vi "Relatorio1LabView.vi"() -> ()   [LabVIEW 2019]
uses:
  <vilib>/Instr/_visa.llb/VISA Configure Serial Port (Instr).vi
  <vilib>/express/express analysis/Spectral/Block/exnSpectralBlock spectral measurements RMS poly.vi
  <vilib>/express/express analysis/Spectral/Block/exnSpectralBlock spectral measurements RMS WFM.vi
  <vilib>/express/express analysis/Spectral/XNode/ExpressSpectralMeasurementsBlockNode.xnode
panel:
  out "Análise espectral da onda - FFT (RMS)":cluster{"f0":dbl, "df":dbl, "magnitude":dbl[]}(graph)
  out "Amplitude do sinal (v) x tempo (s):":waveform(dbl)(graph)
  in  "Parar":bool
  out "Número de \nAmostras":u32 caption="Número de Amostras"
  in  "Número de Blocos de Dados":u32=100 min=1 max=50000 step=1
  in  "Frequencia de Amostragem":dbl=75000.0
  in  "VCC":dbl=5.0
  in  "Resolução":i16=8
  in  "COM Port":refnum<visa-resource-name>
  in  "Baudrate":u32=2000000
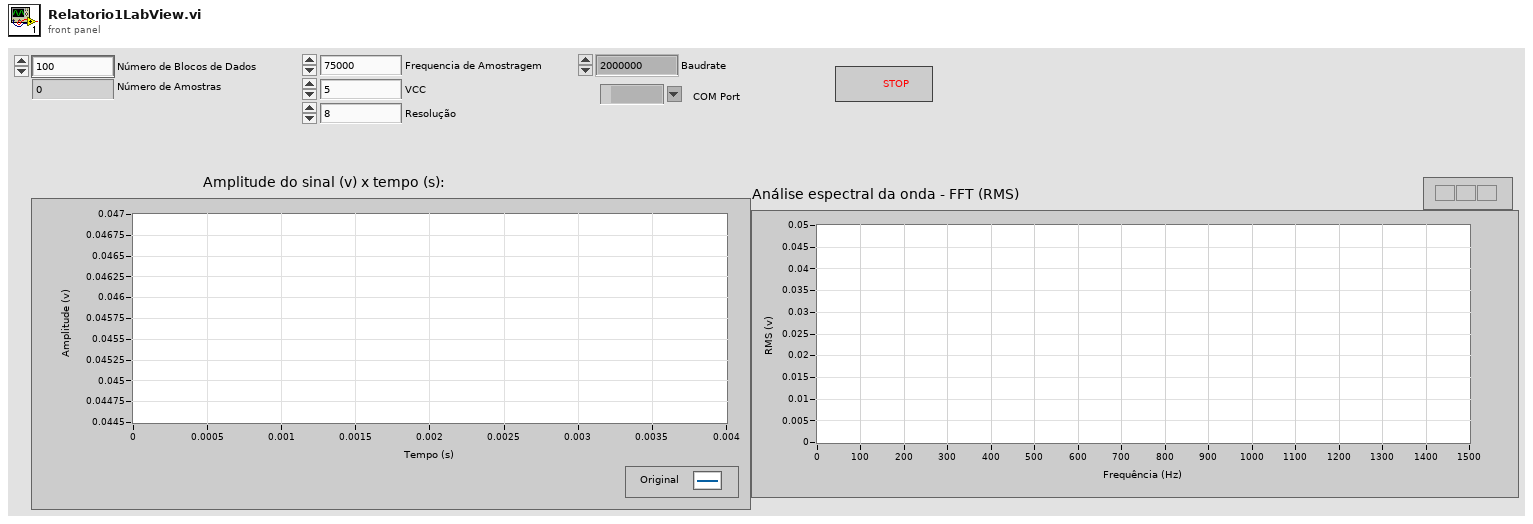
[diagram p1: front panel]
types:
  T1 = cluster{"averaging mode":u16, "weighting mode":u16, "number of averages":u32}
  T2 = cluster{"dB On (F)":bool, "unwrap phase (F)":bool, "convert to degree (F)":bool}
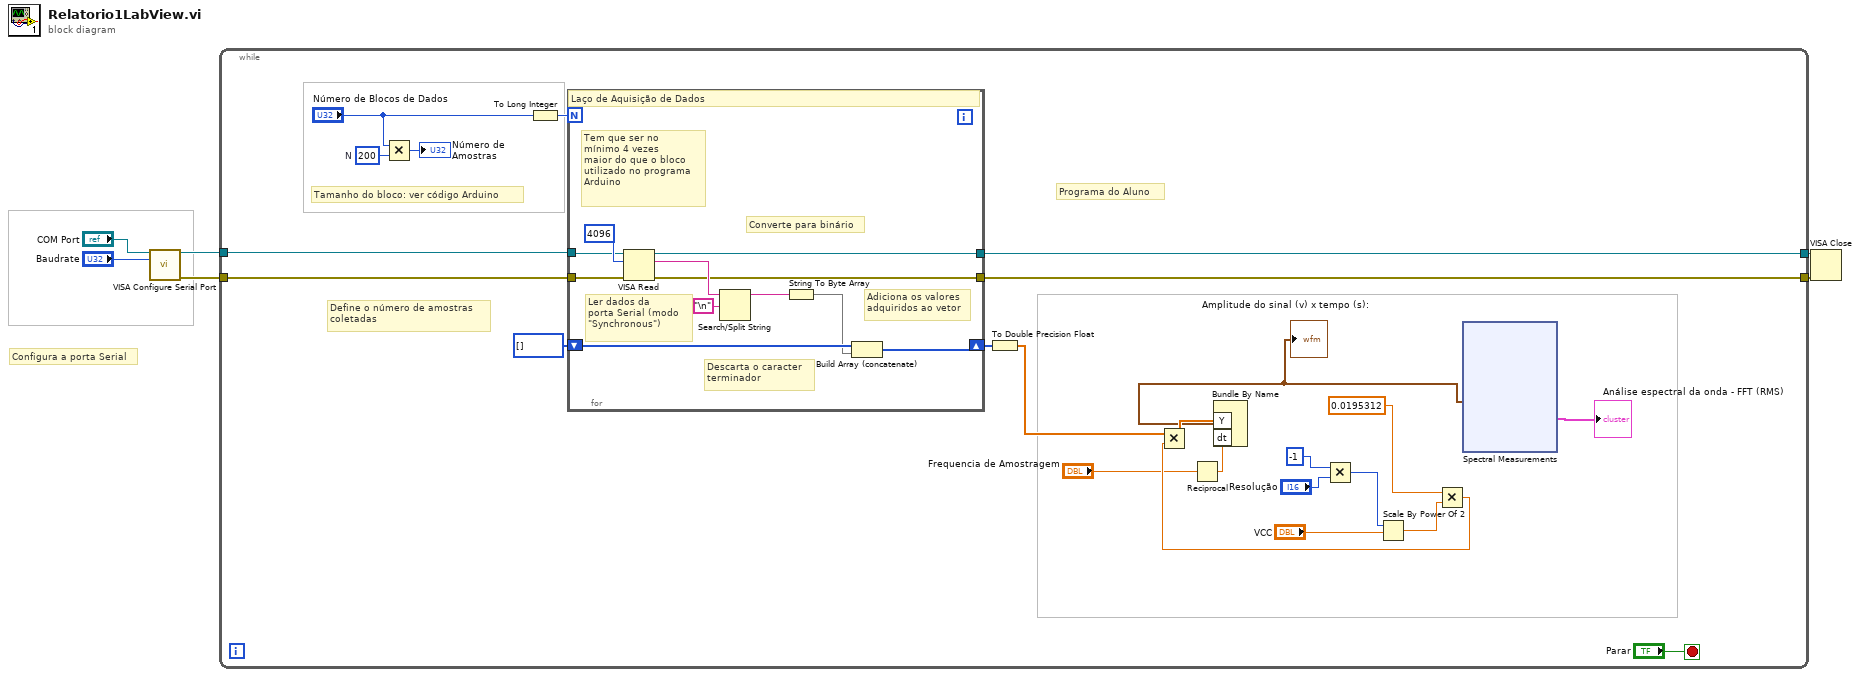
[diagram p0: block diagram]
diagram:
  # "Configura a porta Serial"
  n1 = call-poly "VISA Configure Serial Port"("VISA resource name"="COM Port", "baud rate (9600)"="Baudrate") -> ("VISA resource name out"=w4:refnum<visa-resource-name>, "error out"=w3:errorcluster)  [unwired: 12 in]
  n2 = while {
    tunnel: w4 -> [w30]
    tunnel: w3 -> [w29]
    tunnel: [w28] -> w2
    tunnel: [w27] -> w1
    stop <- "Parar" stop-if-true
    w21 = u32 200  # N
    # "Programa do Aluno"
    # "Tamanho do bloco: ver código Arduino"
    # "Define o número de amostras \ncoletadas"
    n3 = Multiply(x="Número de Blocos de Dados", y=w21) -> (x*y=→"Número de \nAmostras":u32)
    n4 = To Long Integer(number="Número de Blocos de Dados") -> (32bit integer=w24:i32)
    n5 = for {
      N: w24 -> [_]
      tunnel: w30 -> [w47]
      tunnel: w29 -> [w46]
      tunnel: [w45] -> w28
      tunnel: [w44] -> w27
      shift-right: [w41] -> w20
      shift-left: u8[] [] -> [w43]
      # "Adiciona os valores\nadquiridos ao vetor"
      # "Converte para binário"
      # "Descarta o caracter\nterminador"
      # "Ler dados da\nporta Serial (modo \"Synchronous\")"
      # "Tem que ser no \nmínimo 4 vezes \nmaior do que o bloco\nutilizado no programa \nArduino"
      # "Laço de Aquisição de Dados"
      n6 = VISA Read(VISA resource name=w47, byte count=u32 4096, error in (no error)=w46) -> (VISA resource name out=w45:refnum<visa-resource-name>, read buffer=w49:string, error out=w44:errorcluster)  [unwired: 1 out]
      n7 = Search/Split String(string=w49, search string/char (-)="\n") -> (substring before match=w51:string)  [unwired: 1 in, 2 out]
      n8 = String To Byte Array(string=w51) -> (unsigned byte array=w42:u8[])
      n9 = Build Array (concatenate)(w43, w42) -> (w41:u8[])
    }
    n10 = To Double Precision Float(number=w20) -> (double precision float=w19:dbl[])
    n11 = Reciprocal(x="Frequencia de Amostragem") -> (1/x=w7:dbl)
    n12 = Multiply(x=-1, y="Resolução") -> (x*y=w14:i32)
    n13 = Scale By Power Of 2(n=w14, x="VCC") -> (x*2^n=w13:dbl)
    n14 = Multiply(x=0.0195312, y=w13) -> (x*y=w11:dbl)
    n15 = Multiply(x=w19, y=w11) -> (x*y=w18:dbl[])
    n16 = Bundle By Name("Y"=w18, "dt"=w7) -> (w9:waveform(dbl))  [unwired: 1 in]
    "Amplitude do sinal (v) x tempo (s):" <- w9
    n17 = xnode "Spectral Measurements"("Signals"=w9) -> ("FFT - (RMS)"=→"Análise espectral da onda - FFT (RMS)":cluster{"f0":dbl, "df":dbl, "magnitude":dbl[]})  [unwired: 1 in, 2 out]
  }
  n18 = VISA Close(VISA resource name=w2, error in (no error)=w1) -> ()  [unwired: 1 out]
